vi "ValidateModulesConfig.vi"(8 "error in (no error)":errorcluster, 10 "Device":T3, 11 "system info":T1) -> (0 "error out":errorcluster, 2 "description":string, 3 "valid":bool)   [LabVIEW 2017, in "FpgaBitfileManager.lvlib"]
uses:
  <vilib>/addons/InsightCM/Devices/Shared/Common/FpgaBitfileManager/FpgaBitfileManager.lvlib
  <vilib>/addons/InsightCM/MessageBus/Base/controls/R2_Device.ctl
  <vilib>/addons/InsightCM/MessageBus/Base/controls/KeyValuePair.ctl
  <vilib>/addons/InsightCM/MessageBus/Base/controls/DeviceState.ctl
  <vilib>/addons/InsightCM/MessageBus/Base/controls/R2_DataGroup.ctl
  <vilib>/addons/InsightCM/MessageBus/Base/controls/OperatingState.ctl
  <vilib>/addons/InsightCM/MessageBus/Base/controls/Trigger.ctl
  <vilib>/addons/InsightCM/MessageBus/Base/controls/Condition.ctl
  <vilib>/addons/InsightCM/MessageBus/Base/controls/BurstModeTrigger.ctl
  <vilib>/addons/cRIODetectHW/control/SystemHW.ctl
  <vilib>/addons/cRIODetectHW/control/cRIO Product Info.ctl
  <vilib>/addons/cRIODetectHW/cRIODetectHW.lvlib
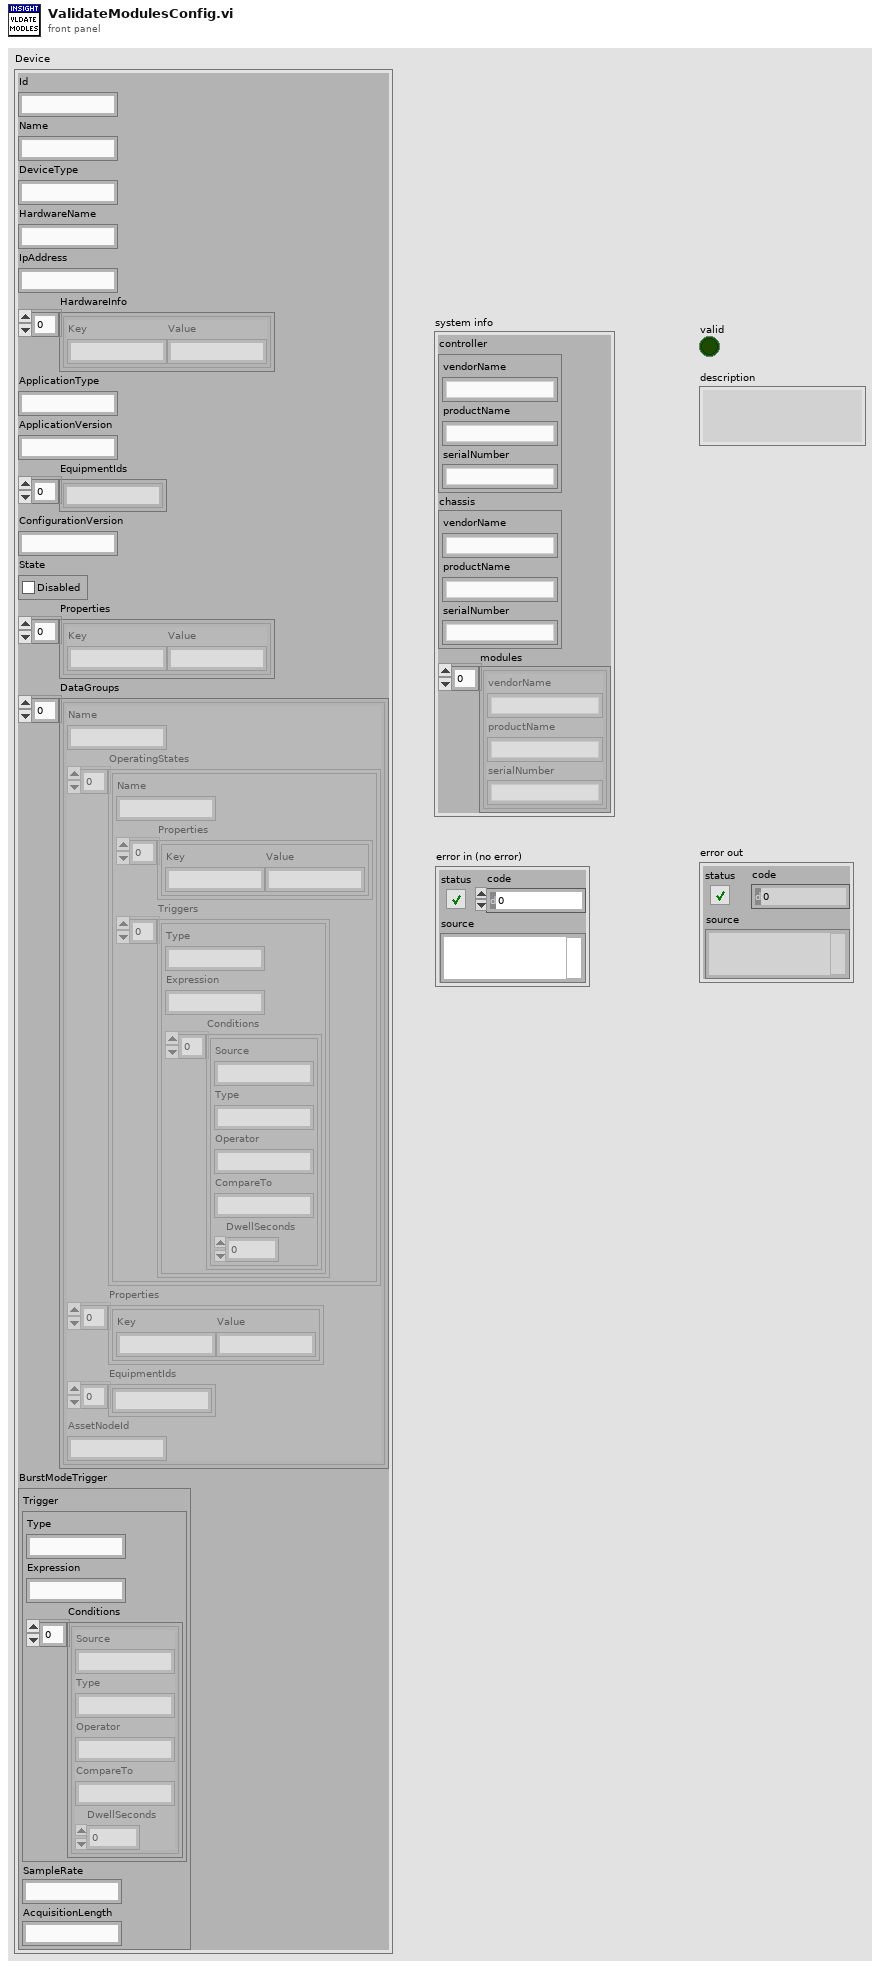
[diagram p1: front panel]
types:
  T1 = typedef "cRIODetectHW.lvlib/SystemHW.ctl" = cluster{"controller":T2, "chassis":T2, "modules":T2[]}
  T2 = typedef "cRIODetectHW.lvlib/cRIO Product Info.ctl" = cluster{"vendorName":string, "productName":string, "serialNumber":string}
  T3 = typedef "R2_Device.ctl" = cluster{"Id":string, "Name":string, "DeviceType":string, "HardwareName":string, "IpAddress":string, "HardwareInfo":T4[], "ApplicationType":string, "ApplicationVersion":string, "EquipmentIds":string[], "ConfigurationVersion":string, "State":T5, "Properties":T4[], "DataGroups":T6[], "BurstModeTrigger":T10}
  T4 = typedef "KeyValuePair.ctl" = cluster{"Key":string, "Value":string}
  T5 = typedef "DeviceState.ctl" = cluster{"Disabled":bool}
  T6 = typedef "R2_DataGroup.ctl" = cluster{"Name":string, "OperatingStates":T7[], "Properties":T4[], "EquipmentIds":string[], "AssetNodeId":string}
  T7 = typedef "OperatingState.ctl" = cluster{"Name":string, "Properties":T4[], "Triggers":T8[]}
  T8 = typedef "Trigger.ctl" = cluster{"Type":string, "Expression":string, "Conditions":T9[]}
  T9 = typedef "Condition.ctl" = cluster{"Source":string, "Type":string, "Operator":string, "CompareTo":string, "DwellSeconds":dbl}
  T10 = typedef "BurstModeTrigger.ctl" = cluster{"Trigger":T8, "SampleRate":string, "AcquisitionLength":string}
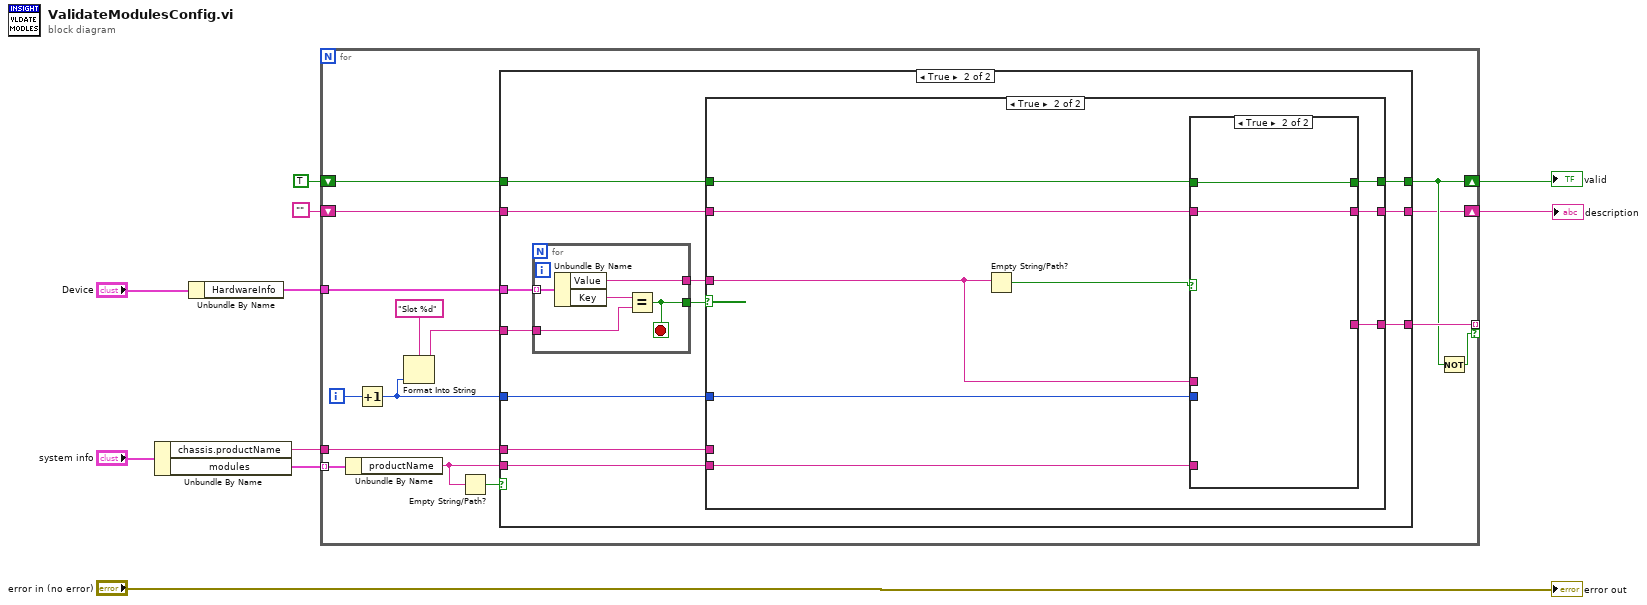
[diagram p0: block diagram]
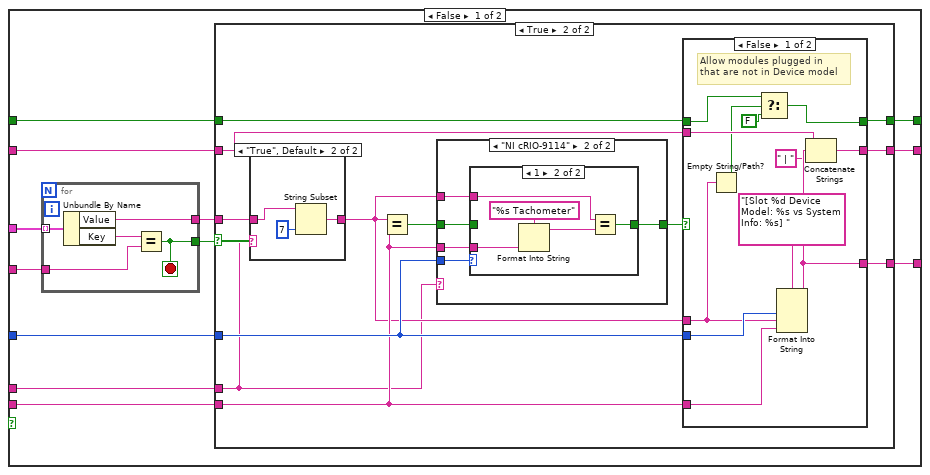
[diagram p2: hidden frame]
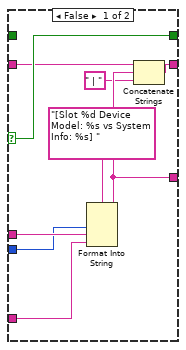
[diagram p9: hidden frame]
diagram:
  n1 = Unbundle By Name("system info") -> ("chassis.productName"=w5:string, "modules"=w9:T2[])
  n2 = Unbundle By Name("Device") -> ("HardwareInfo"=w8:T4[])
  n3 = for {
    tunnel: w8 -> [w21]
    tunnel: w9 -> [w25] mode=indexing
    shift-right: [w16] -> w4
    shift-left: TRUE -> [w19]
    tunnel: [w18] -> _ mode=indexing if=w17
    tunnel: w5 -> [w13]
    shift-right: [w11] -> w1
    shift-left: "" -> [w12]
    i -> [w15]
    n4 = Unbundle By Name(w25) -> ("productName"=w20:string)
    n5 = Increment(x=w15) -> (x+1=w14:i32)
    n6 = Format Into String(format string="Slot %d", w14) -> (resulting string=w22:string)  [unwired: 2 in, 1 out]
    n7 = Empty String/Path?(string/path=w20) -> (empty?=w24:bool)
    n8 = case shown="True" w24 {
      tunnel: w22 -> [w37 w98]
      tunnel: w21 -> [w34 w95]
      tunnel: w20 -> [w33 w94]
      tunnel: [w32 w93] -> w16
      tunnel: w19 -> [w31 w92]
      tunnel: [w30 w91] -> w18
      tunnel: w14 -> [w29 w90]
      tunnel: w13 -> [w28 w89]
      tunnel: w12 -> [w27 w88]
      tunnel: [w26 w87] -> w11
      frame False {
        n9 = for {
          tunnel: w37 -> [w84]
          tunnel: w34 -> [w86] mode=indexing
          tunnel: [w83] -> w36
          tunnel: [w82] -> w35
          stop <- w83 stop-if-true
          n10 = Unbundle By Name(w86) -> ("Value"=w82:string, "Key"=w85:string)
          n11 = Equal?(x=w85, y=w84) -> (x = y?=w83:bool)
        }
        n12 = case shown="True" w36 {
          tunnel: w35 -> [_ w44]
          tunnel: w33 -> [_ w45]
          tunnel: [w39 w51] -> w32
          tunnel: w31 -> [w39 w50]
          tunnel: [_ w49] -> w30
          tunnel: w29 -> [_ w48]
          tunnel: w28 -> [_ w42]
          tunnel: w27 -> [w38 w41]
          tunnel: [w38 w40] -> w26
          frame False {
            # "Physical module detected, but no module\nin the Device Model in this slot. \n\nThis is ok, because it is not a problem to\nhave an unused module in the chassis and\nwe would not want to force people to\nphysically remove unused modules."
          }
          frame True {
            n13 = case shown="\"True\", Default" w42 {
              tunnel: w44 -> [w52 w54]
              tunnel: [w52 w53] -> w43
              frame "NI cRIO-9114" {
              }
              frame "True", Default {
                n14 = String Subset(string=w54, length (rest)=7 ("length (rest)")) -> (substring=w53:string)  [unwired: 1 in]
              }
            }
            n15 = Equal?(x=w43, y=w45) -> (x = y?=w46:bool)
            n16 = case shown="\"NI cRIO-9114\"" w42 {
              tunnel: w48 -> [_ w61]
              tunnel: [w56 w60] -> w47
              tunnel: w46 -> [w56 w59]
              tunnel: w43 -> [_ w58]
              tunnel: w45 -> [_ w57]
              frame Default {
              }
              frame "NI cRIO-9114" {
                n17 = case shown="1" w61 {
                  tunnel: [w62 w65] -> w60
                  tunnel: w59 -> [w62 _]
                  tunnel: w58 -> [_ w63]
                  tunnel: w57 -> [_ w67]
                  frame 0, Default {
                  }
                  frame 1 {
                    n18 = Format Into String(format string="%s Tachometer", w67) -> (resulting string=w64:string)  [unwired: 2 in, 1 out]
                    n19 = Equal?(x=w63, y=w64) -> (x = y?=w65:bool)
                  }
                }
              }
            }
            n20 = case shown="False" w47 {
              tunnel: [w70 w81] -> w51
              tunnel: [w75 _] -> w49
              tunnel: w50 -> [w71 w81]
              tunnel: w45 -> [w73 _]
              tunnel: w43 -> [w69 _]
              tunnel: w48 -> [w79 _]
              tunnel: w41 -> [w77 w80]
              tunnel: [w76 w80] -> w40
              frame False {
                # "Allow modules plugged in\nthat are not in Device model"
                n21 = Empty String/Path?(string/path=w69) -> (empty?=w72:bool)
                n22 = Select(t=w71, s=w72, f=FALSE) -> (s? t:f=w70:bool)
                n23 = Format Into String(format string="[Slot %d Device Model: %s vs System Info: %s] ", w79, w69, w73) -> (resulting string=w75:string)  [unwired: 2 in, 1 out]
                n24 = Concatenate Strings(w77, w75, " | " ("string")) -> (w76:string)
              }
              frame True {
              }
            }
          }
        }
      }
      frame True {
        n25 = for {
          tunnel: w98 -> [w123]
          tunnel: w95 -> [w125] mode=indexing
          tunnel: [w122] -> w97
          tunnel: [w121] -> w96
          stop <- w122 stop-if-true
          n26 = Unbundle By Name(w125) -> ("Value"=w121:string, "Key"=w124:string)
          n27 = Equal?(x=w124, y=w123) -> (x = y?=w122:bool)
        }
        n28 = case shown="True" w97 {
          tunnel: w96 -> [_ w104]
          tunnel: w94 -> [_ w105]
          tunnel: [w100 w109] -> w93
          tunnel: w92 -> [w100 w108]
          tunnel: [_ w107] -> w91
          tunnel: w90 -> [_ w106]
          tunnel: w89 -> [_ _]
          tunnel: w88 -> [w99 w102]
          tunnel: [w99 w101] -> w87
          frame False {
            # "Physical module detected, but no module\nin the Device Model in this slot. \n\nThis is ok, because it is not a problem to\nhave an unused module in the chassis and\nwe would not want to force people to\nphysically remove unused modules."
          }
          frame True {
            n29 = Empty String/Path?(string/path=w104) -> (empty?=w103:bool)
            n30 = case shown="True" w103 {
              selector: w103 -> [w118 _]
              tunnel: [w118 w120] -> w109
              tunnel: [w112 _] -> w107
              tunnel: w108 -> [_ w120]
              tunnel: w105 -> [w117 _]
              tunnel: w104 -> [w116 _]
              tunnel: w106 -> [w115 _]
              tunnel: w102 -> [w113 w119]
              tunnel: [w110 w119] -> w101
              frame False {
                n31 = Format Into String(format string="[Slot %d Device Model: %s vs System Info: %s] ", w115, w116, w117) -> (resulting string=w112:string)  [unwired: 2 in, 1 out]
                n32 = Concatenate Strings(w113, w112, " | ") -> (w110:string)
              }
              frame True {
              }
            }
          }
        }
      }
    }
    n33 = Not(x=w16) -> (.not. x?=w17:bool)
  }
  "valid" <- w4
  "description" <- w1
  "error out" <- "error in (no error)"
